vi "AlGaInPAs_v20b.vi"(2 "Debug Mode":bool, 3 "Elapsed Time(s)":dbl, 4 "State":enum16{"Edit", "Start", "Run", "End", "Idle"}(ring), 5 "Argument List In":string[](array[string])) -> (0 "Status Out":string, 1 "Argument List Out":string[](array[string]))   [LabVIEW 2011]
panel:
  out "source ref array":refnum<vi>[](array[refnum])
  in  "Se bubbler":T1={"Active"=FALSE, "Prep"=FALSE, "Run"=FALSE, "Flow"=0.0, "Dilution"=FALSE, "Calculated"=0, "MFC1 flow"=0.0, "MFC2 flow"=10.0, "MFC3 flow"=100.0} caption="Al" {"MFC1 flow" format="%.4f"; "MFC3 flow" format="%.1f"; "MFC2 flow" format="%.2f"; "Calculated" items=["Flow", "MFC1", "MFC2", "MFC3"]; "Flow" format="%.2f"}
  in  "P bubbler":T2 caption="Al" {"Flow" format="%.2f"}
  in  "As gas":T2 caption="Al" {"Flow" format="%.2f"}
  in  "P gas":T2 caption="Al" {"Flow" format="%.2f"}
  in  "In bubbler":T2 caption="Al" {"Flow" format="%.2f"}
  in  "Ga bubbler":T1={"Active"=FALSE, "Prep"=FALSE, "Run"=FALSE, "Flow"=0.0, "Dilution"=FALSE, "Calculated"=0, "MFC1 flow"=0.0, "MFC2 flow"=10.0, "MFC3 flow"=100.0} caption="Al" {"MFC1 flow" format="%.4f"; "MFC3 flow" format="%.1f"; "MFC2 flow" format="%.2f"; "Calculated" items=["Flow", "MFC1", "MFC2", "MFC3"]; "Flow" format="%.2f"}
  in  "Al bubbler":T2 caption="Al" {"Flow" format="%.2f"}
  in  "Tab Control":T3(tab)
  out "Al Prep":bool caption="Pre-run"
  out "Al Run":bool caption="Run"
  out "Al Flow":dbl caption="Al Flow (0-100 sscm)" format="%.2f"
  out "Ga MFC1 flow":dbl caption="R1 (0-10 sscm)" format="%.4f"
  out "Ga MFC3 flow":dbl=100.0 caption="R3 (0-1000 sscm)" format="%.1f"
  out "Ga MFC2 flow":dbl=10.0 caption="R2 (0-100 sscm)" format="%.2f"
  out "Ga Calculated":u16(ring)=1 caption="Calculated" items=["Ga flow", "MFC1", "MFC2", "MFC3"]
  out "Ga Dilution":bool caption="Dilute"
  out "Ga Prep":bool caption="Pre-run"
  out "Ga Run":bool caption="Run"
  out "Ga Flow":dbl caption="Ga Flow (0-10 sscm)" format="%.2f"
  out "In Prep":bool caption="Pre-run"
  out "In Run":bool caption="Run"
  out "In Flow":dbl caption="In Flow (0-100 sscm)" format="%.2f"
  out "P gas Run":bool caption="Run"
  out "P gas Prep":bool caption="Pre-run"
  out "P gas Flow":dbl caption="PH3 Flow (0-100 sscm)" format="%.2f"
  out "As gas Prep":bool caption="Pre-run"
  out "As gas Run":bool caption="Run"
  out "As gas Flow":dbl caption="AsH3 Flow (0-10 sscm)" format="%.2f"
  out "P liq Prep":bool caption="Pre-run"
  out "P liq Run":bool caption="Run"
  out "P liq Flow":dbl caption="P bubbler Flow (0-100 sscm)" format="%.2f"
  out "Se MFC1 flow":dbl caption="R1 (0-10 sscm)" format="%.4f"
  out "Se MFC3 flow":dbl=100.0 caption="R3 (0-1000 sscm)" format="%.1f"
  out "Se MFC2 flow":dbl=10.0 caption="R2 (0-100 sscm)" format="%.2f"
  out "Se Calculated":u16(ring)=1 caption="Calculated" items=["Ga flow", "MFC1", "MFC2", "MFC3"]
  out "Se Dilution":bool caption="Dilute"
  out "Se Prep":bool caption="Pre-run"
  out "Se Run":bool caption="Run"
  out "Se Flow":dbl caption="Se Flow (0-10 sscm)" format="%.2f"
  out "prep_done":bool
  out "run started":bool
  out "first":bool=TRUE
  out "total time":dbl
  out "is OK?":bool
  in  "prep_time":dbl
  in  "Cancel":bool
  in  "OK":bool
  out "tTotal(s) 2":dbl
  # "s"
  # "Add pre-run time to run time in editor."
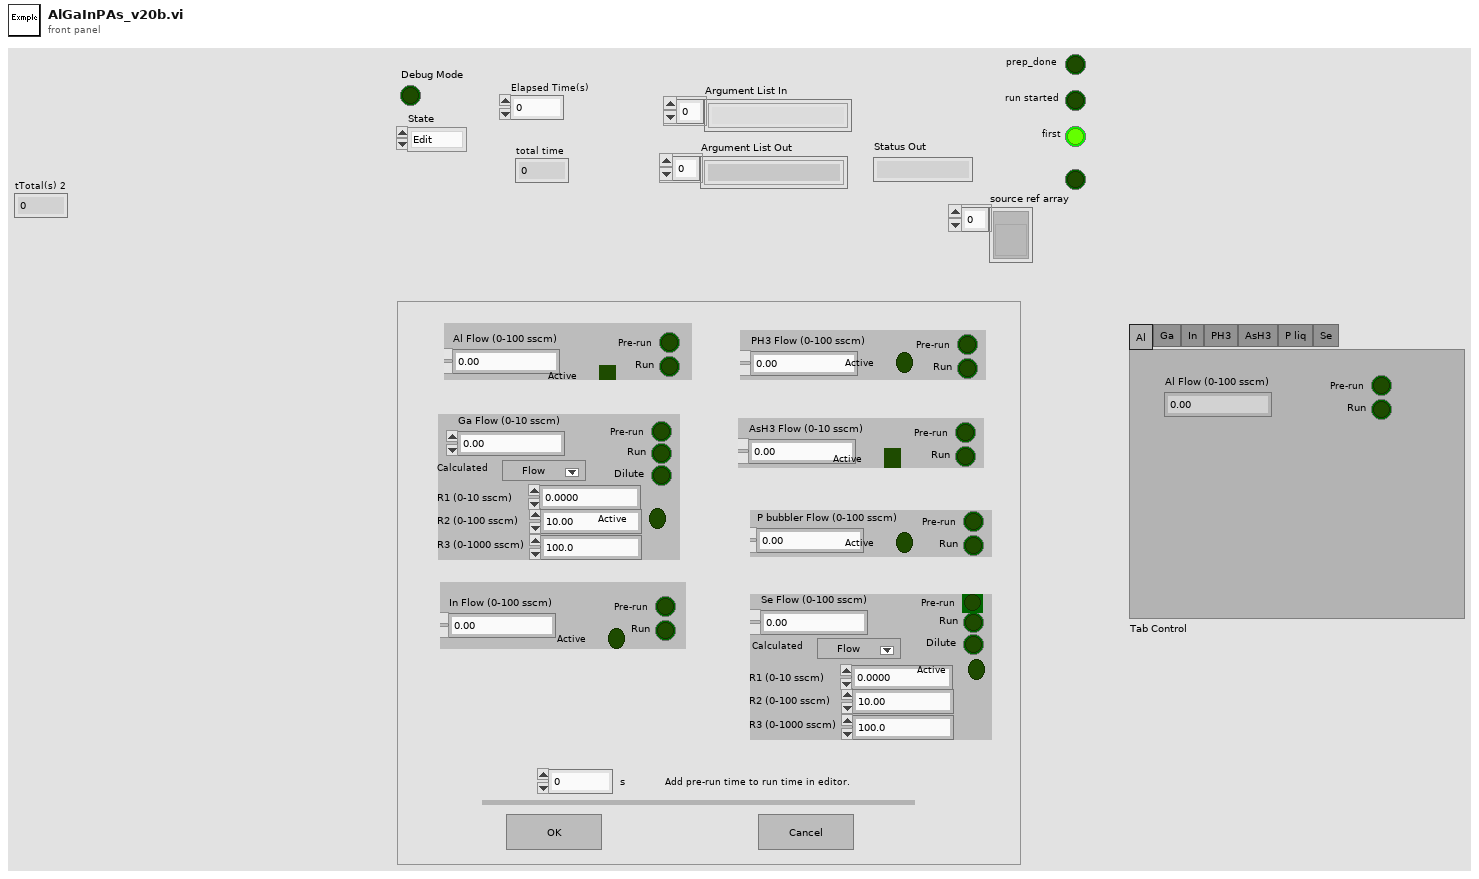
[diagram p1: front panel]
types:
  T1 = cluster{"Active":bool, "Prep":bool, "Run":bool, "Flow":dbl, "Dilution":bool, "Calculated":u16, "MFC1 flow":dbl, "MFC2 flow":dbl, "MFC3 flow":dbl}
  T2 = cluster{"Active":bool, "Prep":bool, "Run":bool, "Flow":dbl}
  T3 = enum32{"Al", "Ga", "In", "PH3", "AsH3", "P liq", "Se"}
  T4 = enum16{"Discrete", "Continuous", "Instantaneous", "Finite"}
  T5 = enum32{"Invalid", "Default", "Floating", "Floating/Auto-Hide", "Modal"}
  T6 = enum8{"Enabled", "Disabled", "Disabled and Grayed Out"}
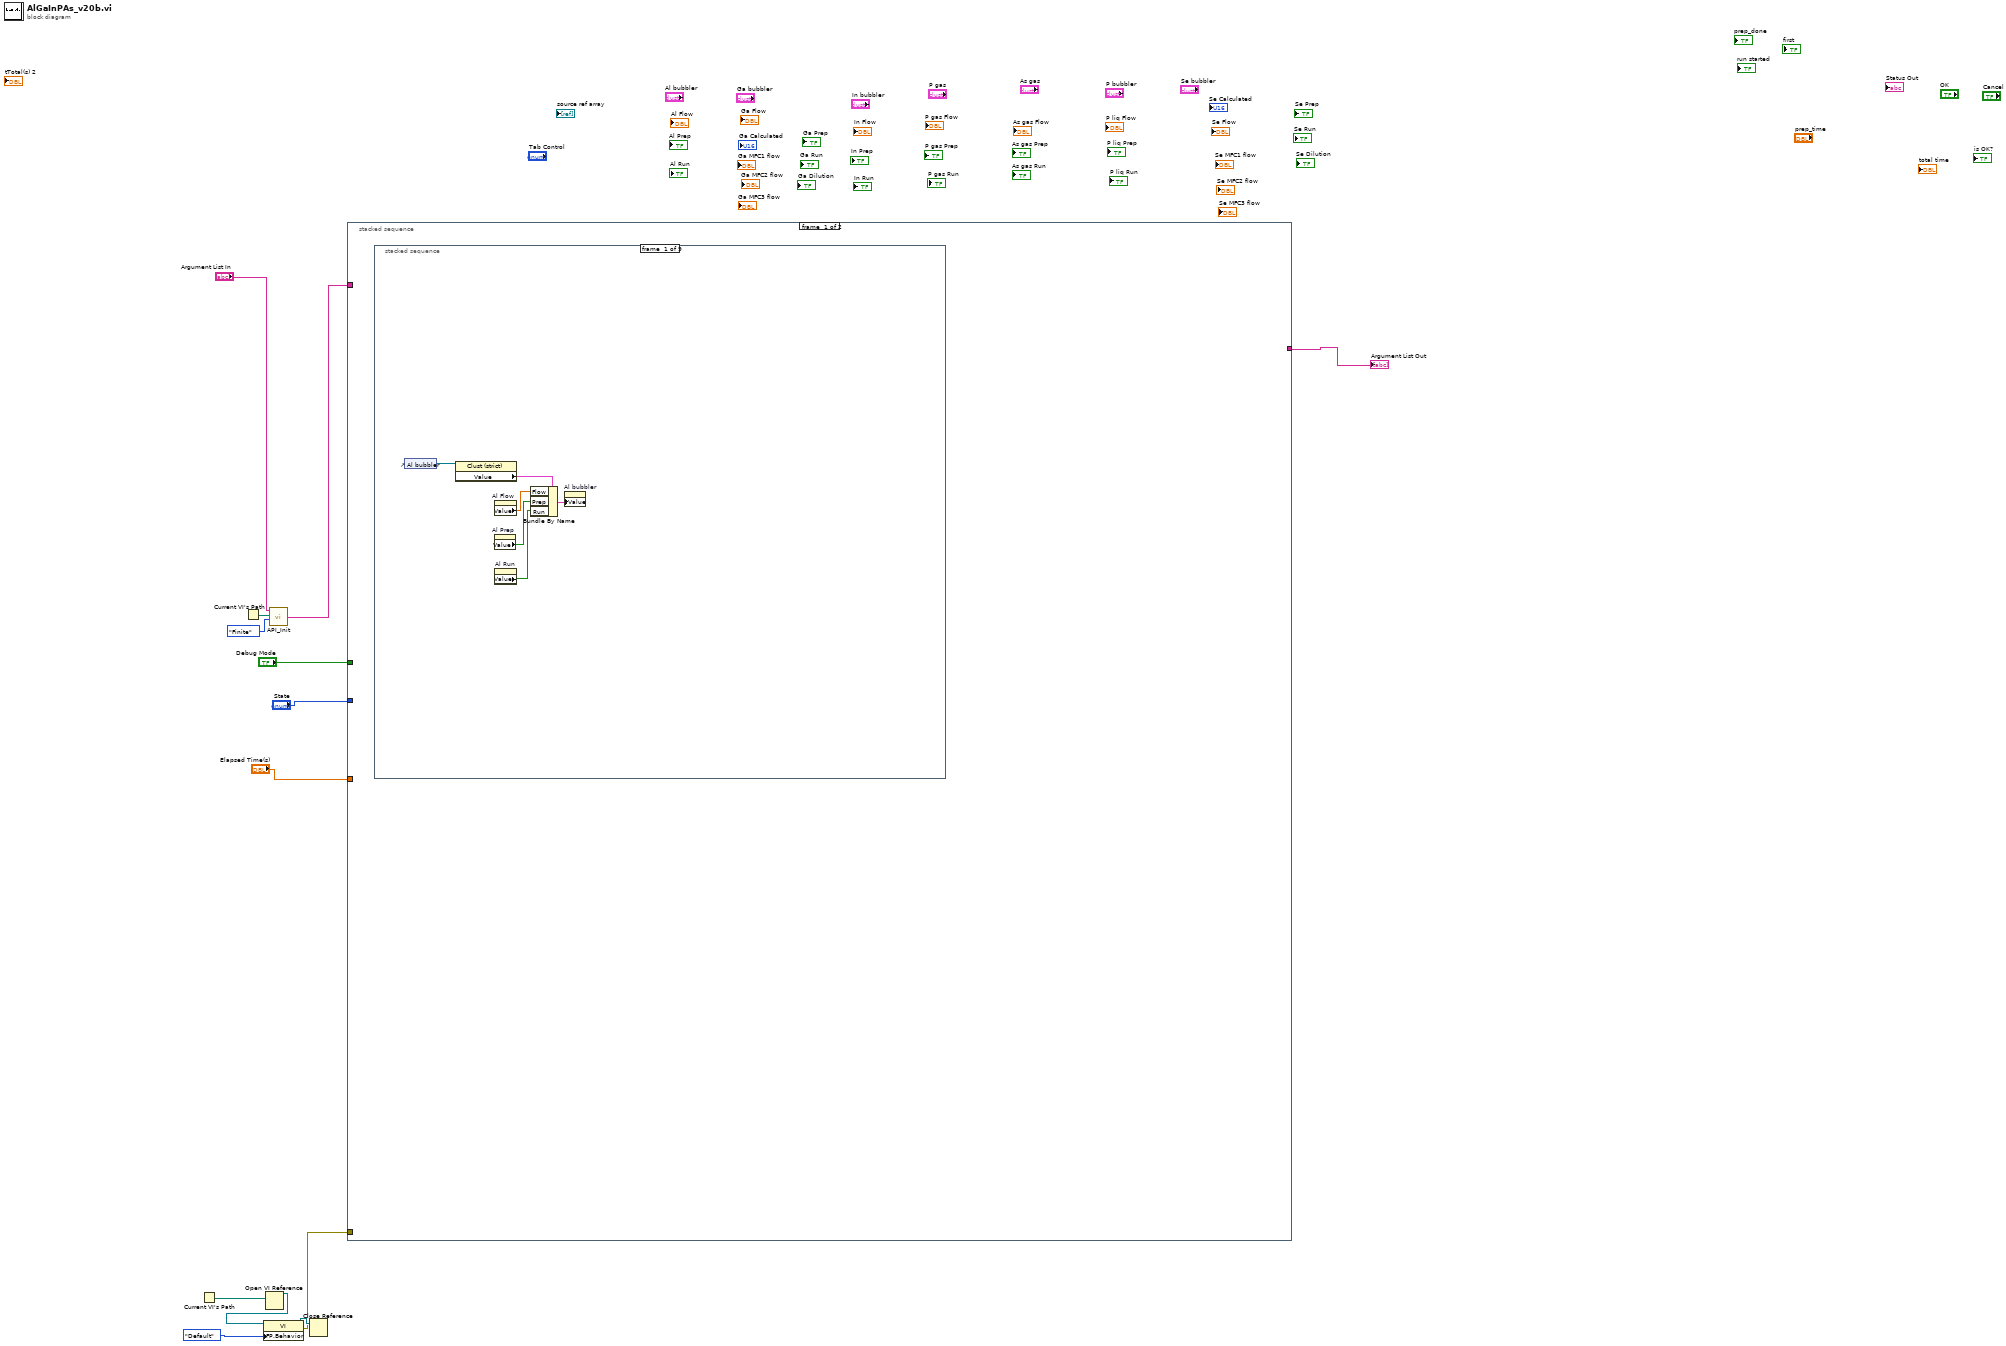
[diagram p0: block diagram]
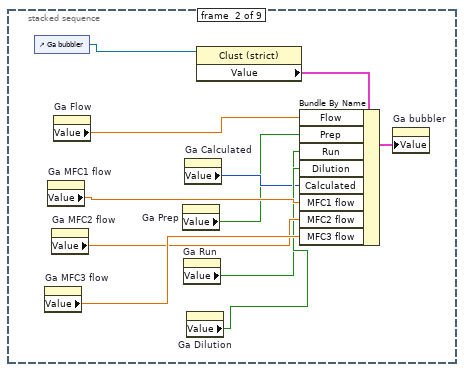
[diagram p2: hidden frame]
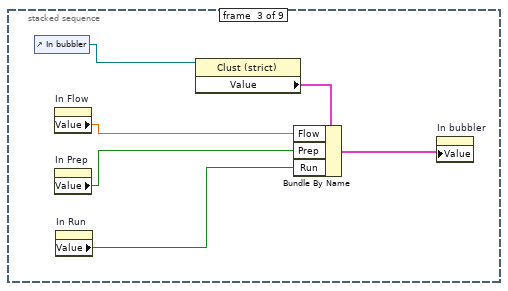
[diagram p3: hidden frame]
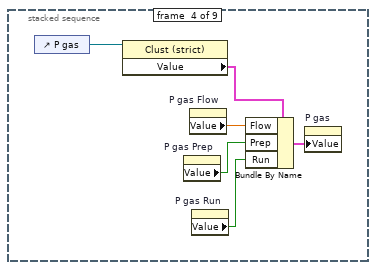
[diagram p4: hidden frame]
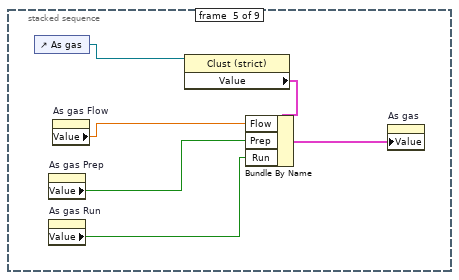
[diagram p5: hidden frame]
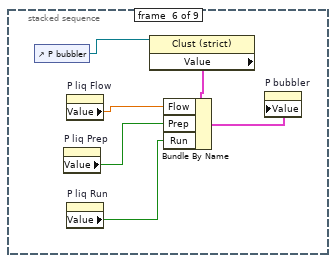
[diagram p6: hidden frame]
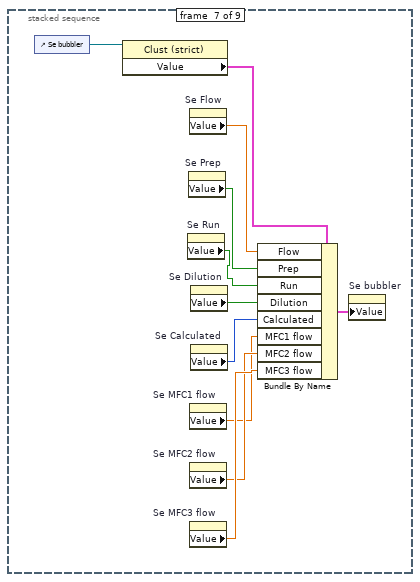
[diagram p7: hidden frame]
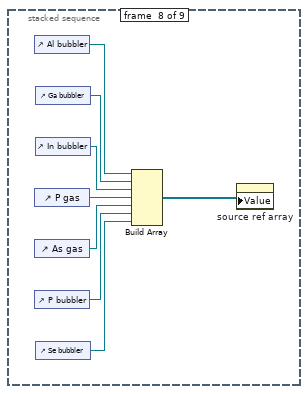
[diagram p8: hidden frame]
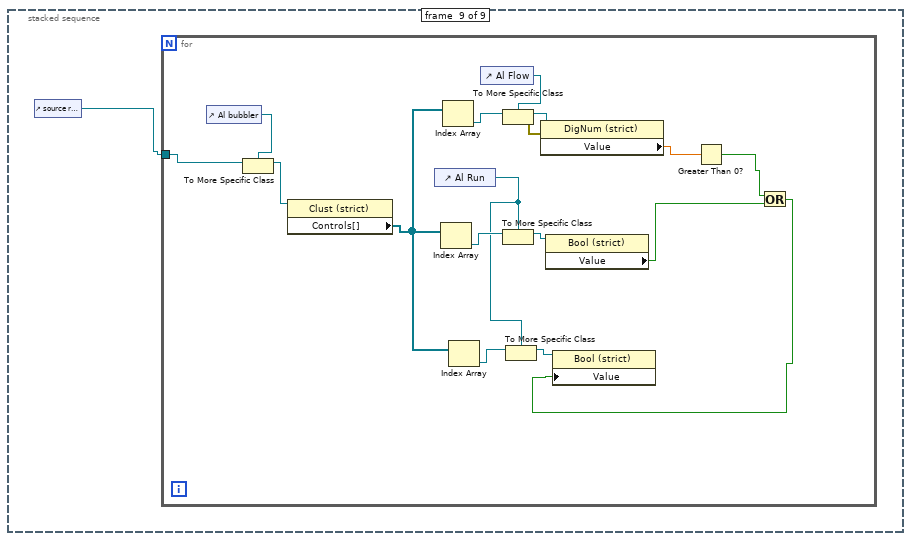
[diagram p9: hidden frame]
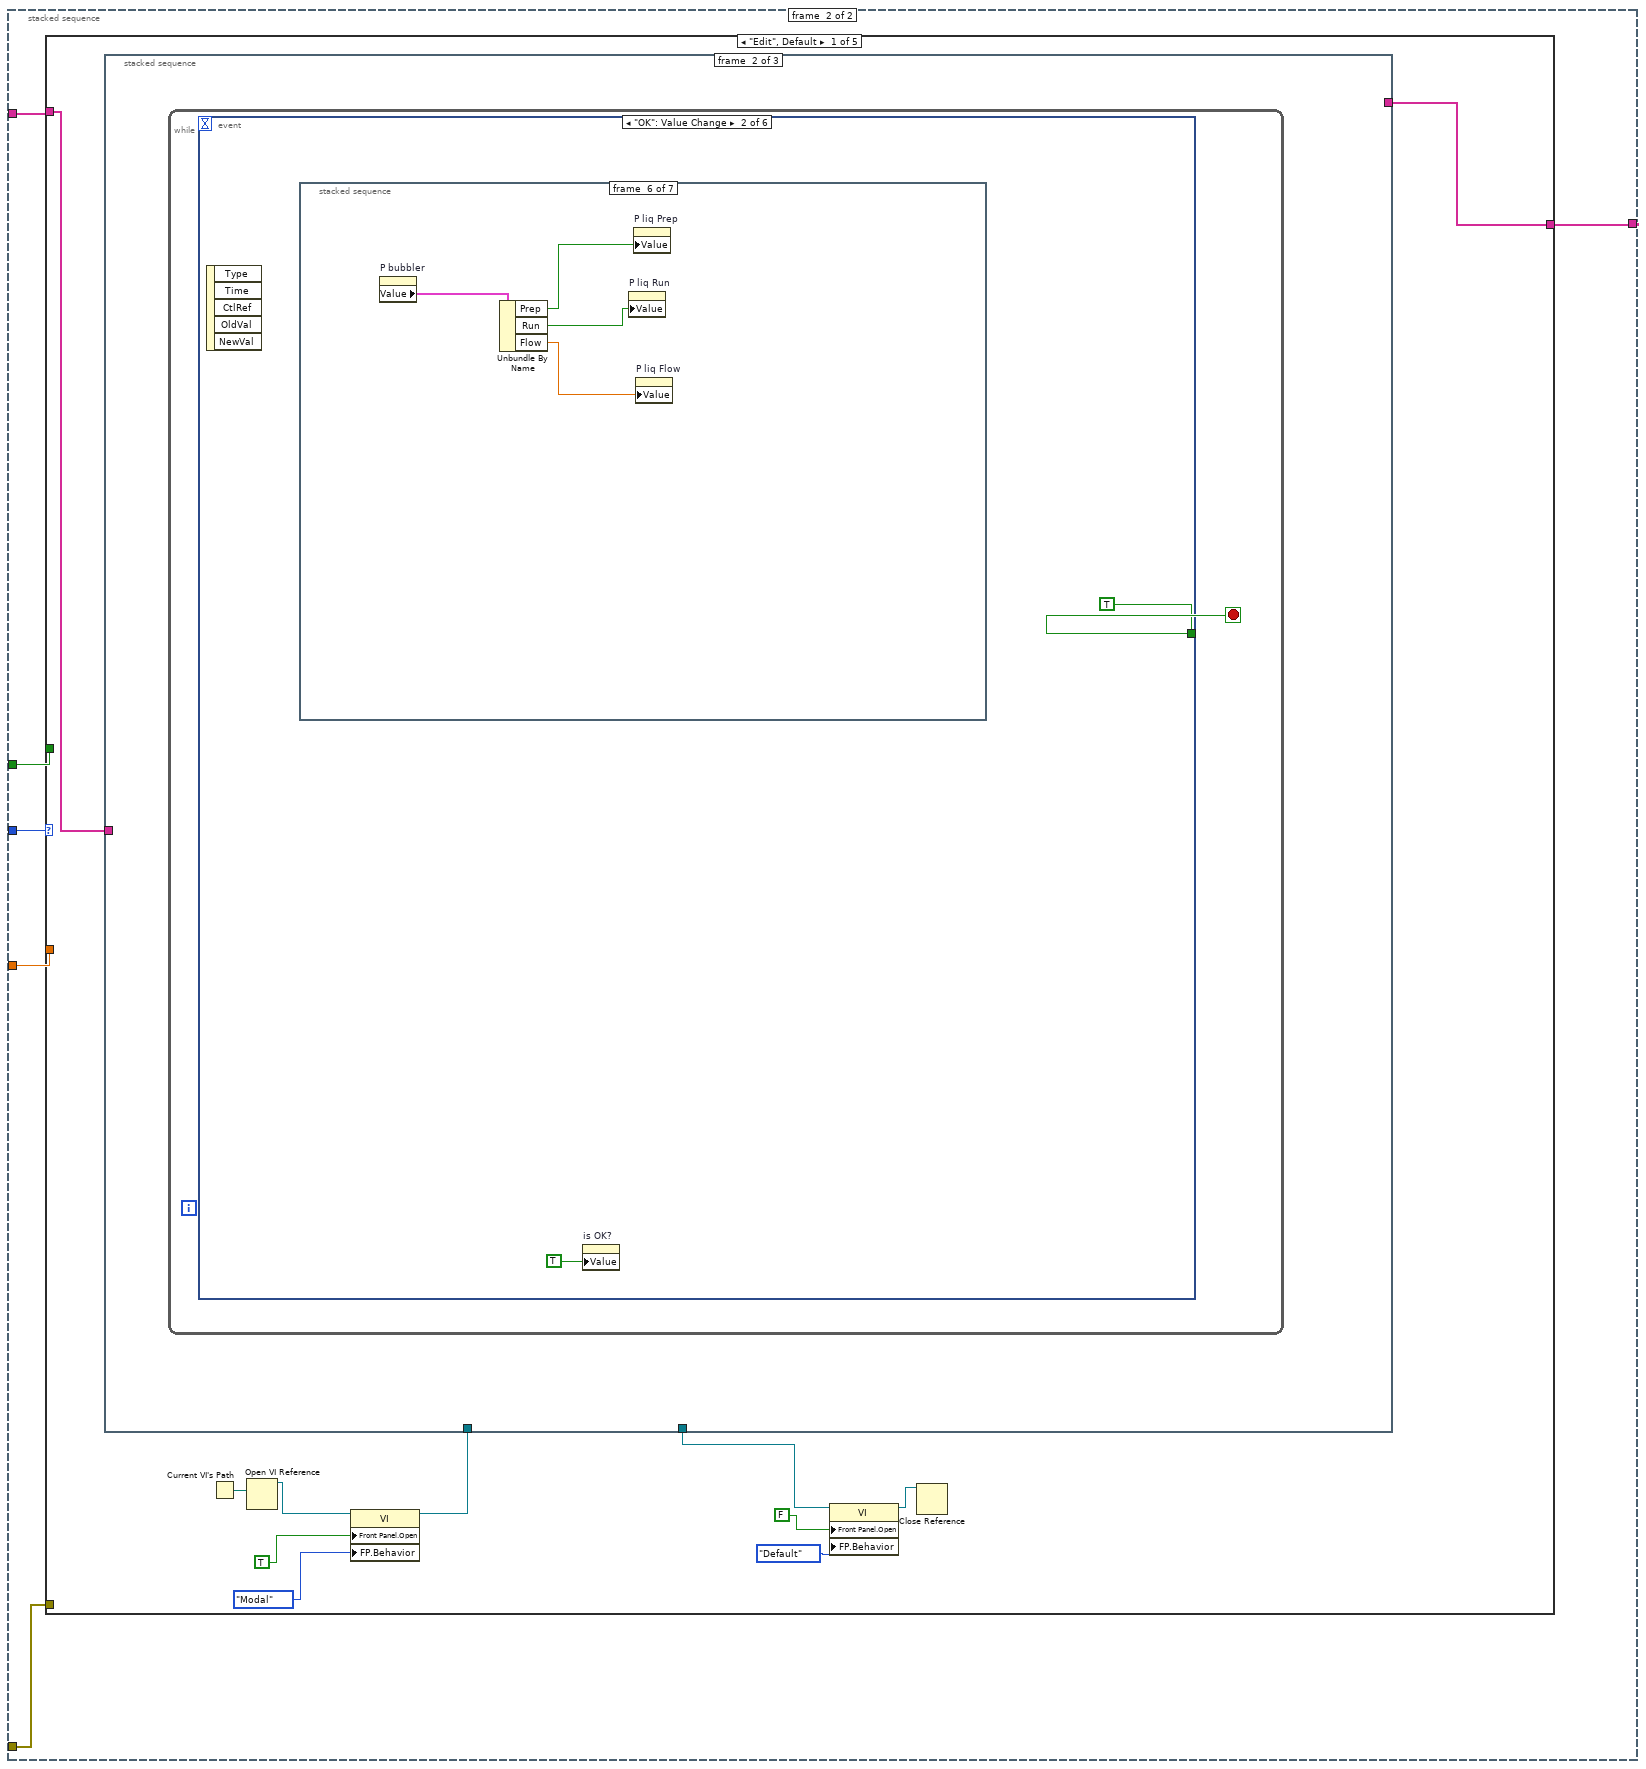
[diagram p10: hidden frame]
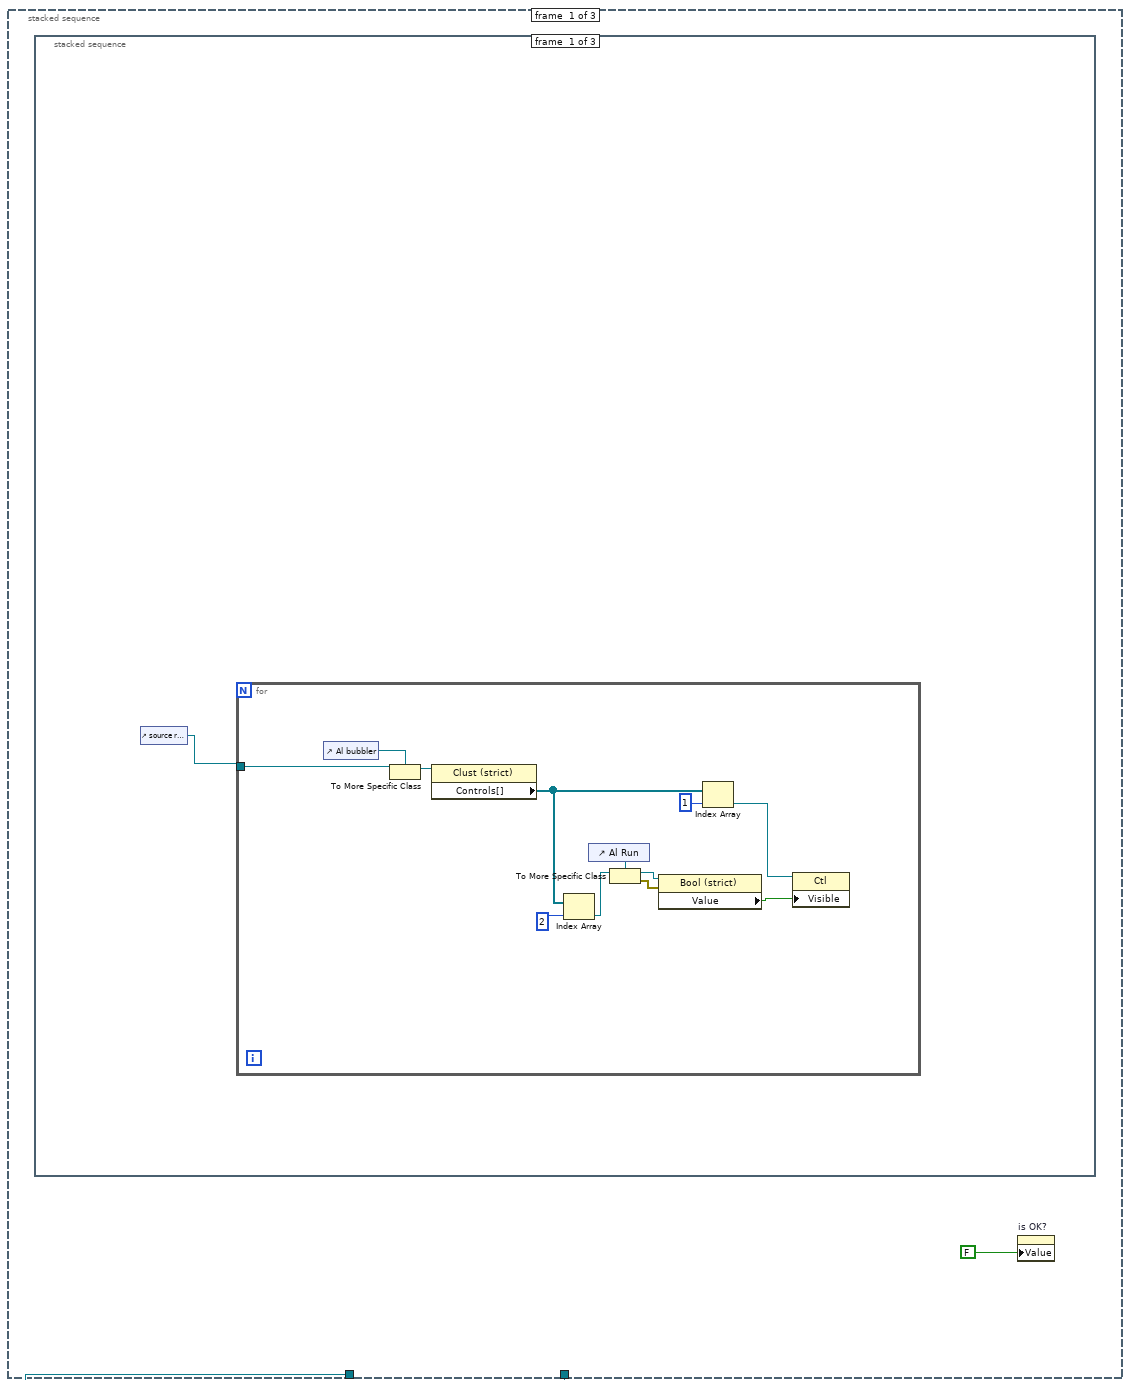
[diagram p11: hidden frame]
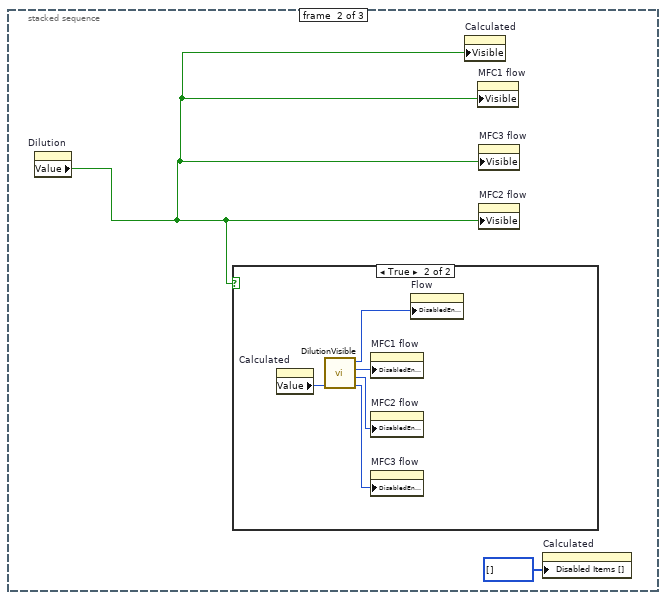
[diagram p12: hidden frame]
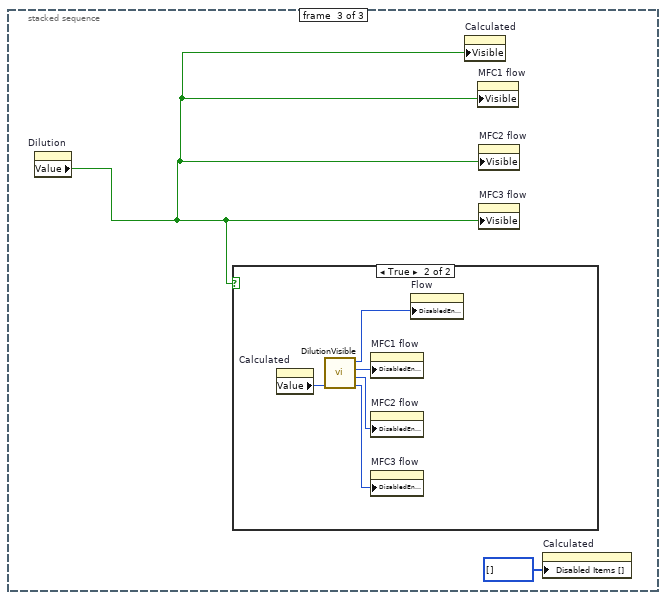
[diagram p14: hidden frame]
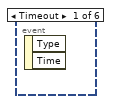
[diagram p16: hidden frame]
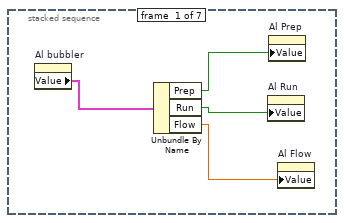
[diagram p17: hidden frame]
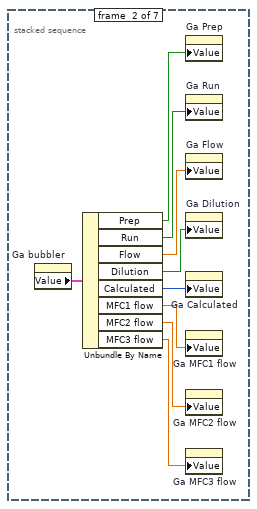
[diagram p18: hidden frame]
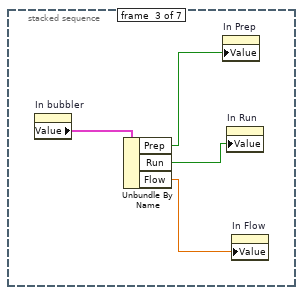
[diagram p19: hidden frame]
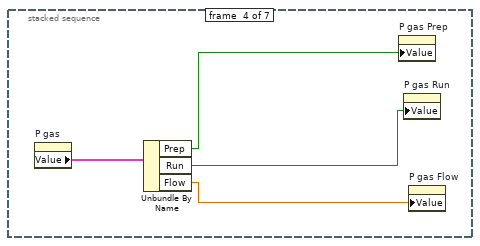
[diagram p20: hidden frame]
diagram:
  n1 = Current VI's Path() -> (path=w9:path)
  n2 = Current VI's Path() -> (path=w4:path)
  n3 = Open VI Reference(vi path=w9) -> (vi reference=w8:refnum<vi>)  [unwired: 1 in, 5 out]
  n4 = property class="VI"(reference=w8, "FP.Behavior"=T5."Default" ("Front Panel Window:Behavior")) -> (reference out=w6:refnum<vi>, error out=w5:errorcluster)  [unwired: 1 in]
  n5 = call "API_Init.vi"("API Mode"=T4."Finite", "VI Path"=w4, "Argument List In"="Argument List In") -> ("Argument List Out"=w1:string[])  [unwired: 1 in]
  n6 = Close Reference(reference=w6) -> ()  [unwired: 1 in, 1 out]
  n7 = stacked-sequence {
    tunnel: "State" -> [_ w97]
    tunnel: "Debug Mode" -> [_ w96]
    tunnel: "Elapsed Time(s)" -> [_ w95]
    tunnel: [_ w94] -> w10
    tunnel: w5 -> [_ w93]
    tunnel: w1 -> [_ w92]
    frame #0 {
      n8 = stacked-sequence {
        frame #0 {
          n9 = control-ref of="Al bubbler"() -> (w19:refnum<vi>)
          n10 = property class="Clust (strict)"(reference=w19) -> ("Value"=w18:T2)  [unwired: 1 in, 2 out]
          n11 = property on="Al Prep" class="Bool (strict)"() -> ("Value"=w16:bool)  [unwired: 2 in, 2 out]
          n12 = property on="Al Flow" class="DigNum (strict)"() -> ("Value"=w17:dbl)  [unwired: 2 in, 2 out]
          n13 = property on="Al Run" class="Bool (strict)"() -> ("Value"=w15:bool)  [unwired: 2 in, 2 out]
          n14 = Bundle By Name(cluster=w18, "Flow"=w17, "Prep"=w16, "Run"=w15) -> (w14:T2)
          n15 = property on="Al bubbler" class="Clust (strict)"("Value"=w14) -> ()  [unwired: 2 in, 2 out]
        }
        frame #1 {
          n16 = control-ref of="Ga bubbler"() -> (w20:refnum<vi>)
          n17 = property on="Ga MFC3 flow" class="DigNum (strict)"() -> ("Value"=w30:dbl)  [unwired: 2 in, 2 out]
          n18 = property on="Ga MFC1 flow" class="DigNum (strict)"() -> ("Value"=w28:dbl)  [unwired: 2 in, 2 out]
          n19 = property on="Ga MFC2 flow" class="DigNum (strict)"() -> ("Value"=w29:dbl)  [unwired: 2 in, 2 out]
          n20 = property on="Ga Flow" class="DigNum (strict)"() -> ("Value"=w23:dbl)  [unwired: 2 in, 2 out]
          n21 = property on="Ga Prep" class="Bool (strict)"() -> ("Value"=w24:bool)  [unwired: 2 in, 2 out]
          n22 = property on="Ga Run" class="Bool (strict)"() -> ("Value"=w26:bool)  [unwired: 2 in, 2 out]
          n23 = property on="Ga Calculated" class="Ring (strict)"() -> ("Value"=w25:u16)  [unwired: 2 in, 2 out]
          n24 = property on="Ga Dilution" class="Bool (strict)"() -> ("Value"=w27:bool)  [unwired: 2 in, 2 out]
          n25 = property class="Clust (strict)"(reference=w20) -> ("Value"=w21:T1)  [unwired: 1 in, 2 out]
          n26 = Bundle By Name(cluster=w21, "Flow"=w23, "Prep"=w24, "Run"=w26, "Dilution"=w27, "Calculated"=w25, "MFC1 flow"=w28, "MFC2 flow"=w29, "MFC3 flow"=w30) -> (w22:T1)
          n27 = property on="Ga bubbler" class="Clust (strict)"("Value"=w22) -> ()  [unwired: 2 in, 2 out]
        }
        frame #2 {
          n28 = control-ref of="In bubbler"() -> (w31:refnum<vi>)
          n29 = property on="In Flow" class="DigNum (strict)"() -> ("Value"=w33:dbl)  [unwired: 2 in, 2 out]
          n30 = property on="In Prep" class="Bool (strict)"() -> ("Value"=w35:bool)  [unwired: 2 in, 2 out]
          n31 = property on="In Run" class="Bool (strict)"() -> ("Value"=w36:bool)  [unwired: 2 in, 2 out]
          n32 = property class="Clust (strict)"(reference=w31) -> ("Value"=w32:T2)  [unwired: 1 in, 2 out]
          n33 = Bundle By Name(cluster=w32, "Flow"=w33, "Prep"=w35, "Run"=w36) -> (w34:T2)
          n34 = property on="In bubbler" class="Clust (strict)"("Value"=w34) -> ()  [unwired: 2 in, 2 out]
        }
        frame #3 {
          n35 = control-ref of="P gas"() -> (w37:refnum<vi>)
          n36 = property class="Clust (strict)"(reference=w37) -> ("Value"=w38:T2)  [unwired: 1 in, 2 out]
          n37 = property on="P gas Prep" class="Bool (strict)"() -> ("Value"=w41:bool)  [unwired: 2 in, 2 out]
          n38 = property on="P gas Flow" class="DigNum (strict)"() -> ("Value"=w39:dbl)  [unwired: 2 in, 2 out]
          n39 = property on="P gas Run" class="Bool (strict)"() -> ("Value"=w42:bool)  [unwired: 2 in, 2 out]
          n40 = Bundle By Name(cluster=w38, "Flow"=w39, "Prep"=w41, "Run"=w42) -> (w40:T2)
          n41 = property on="P gas" class="Clust (strict)"("Value"=w40) -> ()  [unwired: 2 in, 2 out]
        }
        frame #4 {
          n42 = control-ref of="As gas"() -> (w44:refnum<vi>)
          n43 = property on="As gas Prep" class="Bool (strict)"() -> ("Value"=w47:bool)  [unwired: 2 in, 2 out]
          n44 = property on="As gas Run" class="Bool (strict)"() -> ("Value"=w48:bool)  [unwired: 2 in, 2 out]
          n45 = property on="As gas Flow" class="DigNum (strict)"() -> ("Value"=w46:dbl)  [unwired: 2 in, 2 out]
          n46 = property class="Clust (strict)"(reference=w44) -> ("Value"=w43:T2)  [unwired: 1 in, 2 out]
          n47 = Bundle By Name(cluster=w43, "Flow"=w46, "Prep"=w47, "Run"=w48) -> (w45:T2)
          n48 = property on="As gas" class="Clust (strict)"("Value"=w45) -> ()  [unwired: 2 in, 2 out]
        }
        frame #5 {
          n49 = control-ref of="P bubbler"() -> (w49:refnum<vi>)
          n50 = property on="P liq Prep" class="Bool (strict)"() -> ("Value"=w53:bool)  [unwired: 2 in, 2 out]
          n51 = property on="P liq Flow" class="DigNum (strict)"() -> ("Value"=w52:dbl)  [unwired: 2 in, 2 out]
          n52 = property on="P liq Run" class="Bool (strict)"() -> ("Value"=w54:bool)  [unwired: 2 in, 2 out]
          n53 = property class="Clust (strict)"(reference=w49) -> ("Value"=w50:T2)  [unwired: 1 in, 2 out]
          n54 = Bundle By Name(cluster=w50, "Flow"=w52, "Prep"=w53, "Run"=w54) -> (w51:T2)
          n55 = property on="P bubbler" class="Clust (strict)"("Value"=w51) -> ()  [unwired: 2 in, 2 out]
        }
        frame #6 {
          n56 = control-ref of="Se bubbler"() -> (w55:refnum<vi>)
          n57 = property class="Clust (strict)"(reference=w55) -> ("Value"=w56:T1)  [unwired: 1 in, 2 out]
          n58 = property on="Se Run" class="Bool (strict)"() -> ("Value"=w60:bool)  [unwired: 2 in, 2 out]
          n59 = property on="Se Prep" class="Bool (strict)"() -> ("Value"=w59:bool)  [unwired: 2 in, 2 out]
          n60 = property on="Se Flow" class="DigNum (strict)"() -> ("Value"=w58:dbl)  [unwired: 2 in, 2 out]
          n61 = property on="Se MFC1 flow" class="DigNum (strict)"() -> ("Value"=w63:dbl)  [unwired: 2 in, 2 out]
          n62 = property on="Se MFC2 flow" class="DigNum (strict)"() -> ("Value"=w64:dbl)  [unwired: 2 in, 2 out]
          n63 = property on="Se MFC3 flow" class="DigNum (strict)"() -> ("Value"=w65:dbl)  [unwired: 2 in, 2 out]
          n64 = property on="Se Dilution" class="Bool (strict)"() -> ("Value"=w61:bool)  [unwired: 2 in, 2 out]
          n65 = property on="Se Calculated" class="Ring (strict)"() -> ("Value"=w62:u16)  [unwired: 2 in, 2 out]
          n66 = Bundle By Name(cluster=w56, "Flow"=w58, "Prep"=w59, "Run"=w60, "Dilution"=w61, "Calculated"=w62, "MFC1 flow"=w63, "MFC2 flow"=w64, "MFC3 flow"=w65) -> (w57:T1)
          n67 = property on="Se bubbler" class="Clust (strict)"("Value"=w57) -> ()  [unwired: 2 in, 2 out]
        }
        frame #7 {
          n68 = control-ref of="Al bubbler"() -> (w73:refnum<vi>)
          n69 = control-ref of="P gas"() -> (w70:refnum<vi>)
          n70 = control-ref of="As gas"() -> (w69:refnum<vi>)
          n71 = control-ref of="P bubbler"() -> (w68:refnum<vi>)
          n72 = control-ref of="Ga bubbler"() -> (w72:refnum<vi>)
          n73 = control-ref of="In bubbler"() -> (w71:refnum<vi>)
          n74 = control-ref of="Se bubbler"() -> (w67:refnum<vi>)
          n75 = Build Array(w73, w72, w71, w70, w69, w68, w67) -> (w66:refnum<vi>[])
          n76 = property on="source ref array" class="Arr (strict)"("Value"=w66) -> ()  [unwired: 2 in, 2 out]
        }
        frame #8 {
          n77 = control-ref of="source ref array"() -> (w74:refnum<vi>)
          n78 = for {
            tunnel: w74 -> [w90]
            n79 = control-ref of="Al bubbler"() -> (w89:refnum<vi>)
            n80 = To More Specific Class(target class=w89, reference=w90) -> (specific class reference=w88:refnum<vi>)  [unwired: 1 in, 1 out]
            n81 = property class="Clust (strict)"(reference=w88) -> ("Controls[]"=w87:refnum<vi>[])  [unwired: 1 in, 2 out]
            n82 = control-ref of="Al Run"() -> (w84:refnum<vi>)
            n83 = Index Array(array=w87) -> (element=w86:refnum<vi>)  [unwired: 1 in]
            n84 = Index Array(array=w87) -> (element=w83:refnum<vi>)  [unwired: 1 in]
            n85 = Index Array(array=w87) -> (element=w85:refnum<vi>)  [unwired: 1 in]
            n86 = control-ref of="Al Flow"() -> (w82:refnum<vi>)
            n87 = To More Specific Class(target class=w82, reference=w83) -> (specific class reference=w79:refnum<vi>, error out=w78:errorcluster)  [unwired: 1 in]
            n88 = To More Specific Class(target class=w84, reference=w86) -> (specific class reference=w81:refnum<vi>)  [unwired: 1 in, 1 out]
            n89 = To More Specific Class(target class=w84, reference=w85) -> (specific class reference=w80:refnum<vi>)  [unwired: 1 in, 1 out]
            n90 = property class="DigNum (strict)"(reference=w79, error in=w78) -> ("Value"=w77:dbl)  [unwired: 2 out]
            n91 = property class="Bool (strict)"(reference=w81) -> ("Value"=w76:bool)  [unwired: 1 in, 2 out]
            n92 = Greater Than 0?(x=w77) -> (x > 0?=w91:bool)
            n93 = Or(x=w91, y=w76) -> (x .or. y?=w75:bool)
            n94 = property class="Bool (strict)"(reference=w80, "Value"=w75) -> ()  [unwired: 1 in, 2 out]
          }
        }
      }
    }
    frame #1 {
      n95 = case shown="\"Edit\", Default" w97 {
        tunnel: w96 -> [_ w235 w247 _ _]
        tunnel: w95 -> [_ _ w248 _ _]
        tunnel: w92 -> [w99 w240 w246 w343 w344]
        tunnel: [w98 w239 w245 w343 w344] -> w94
        tunnel: w93 -> [_ _ _ _ _]
        frame "Edit", Default {
          n96 = Current VI's Path() -> (path=w104:path)
          n97 = Open VI Reference(vi path=w104) -> (vi reference=w103:refnum<vi>)  [unwired: 1 in, 5 out]
          n98 = property class="VI"(reference=w103, "Front Panel.Open"=TRUE ("Front Panel Window:Open"), "FP.Behavior"=T5."Modal" ("Front Panel Window:Behavior")) -> (reference out=w102:refnum<vi>)  [unwired: 1 in, 1 out]
          n99 = stacked-sequence {
            tunnel: w99 -> [_ _ w230]
            tunnel: w102 -> [w110 _ _]
            tunnel: [w110 _ _] -> w106
            tunnel: [_ _ w231] -> w98
            frame #0 {
              n100 = stacked-sequence {
                frame #0 {
                  n101 = control-ref of="source ref array"() -> (w111:refnum<vi>)
                  n102 = for {
                    tunnel: w111 -> [w123]
                    n103 = control-ref of="Al bubbler"() -> (w122:refnum<vi>)
                    n104 = To More Specific Class(target class=w122, reference=w123) -> (specific class reference=w119:refnum<vi>)  [unwired: 1 in, 1 out]
                    n105 = property class="Clust (strict)"(reference=w119) -> ("Controls[]"=w118:refnum<vi>[])  [unwired: 1 in, 2 out]
                    n106 = Index Array(array=w118, index=2) -> (element=w115:refnum<vi>)
                    n107 = control-ref of="Al Run"() -> (w116:refnum<vi>)
                    n108 = To More Specific Class(target class=w116, reference=w115) -> (specific class reference=w114:refnum<vi>, error out=w113:errorcluster)  [unwired: 1 in]
                    n109 = property class="Bool (strict)"(reference=w114, error in=w113) -> ("Value"=w112:bool)  [unwired: 2 out]
                    n110 = Index Array(array=w118, index=1) -> (element=w120:refnum<vi>)
                    n111 = property class="Ctl"(reference=w120, "Visible"=w112) -> ()  [unwired: 1 in, 2 out]
                  }
                }
                frame #1 {
                  n112 = property on="Dilution" class="Bool (strict)"() -> ("Value"=w125:bool)  [unwired: 2 in, 2 out]
                  n113 = case shown="True" w125 {
                    frame False {
                    }
                    frame True {
                      n114 = property on="Calculated" class="Ring (strict)"() -> ("Value"=w126:u16)  [unwired: 2 in, 2 out]
                      n115 = call "DilutionVisible.vi"("calculated"=w126) -> ("MFC3"=w129:u16, "MFC2"=w128:u16, "MFC1"=w127:u16, "flow"=w130:u16)  [unwired: 3 in]
                      n116 = property on="MFC1 flow" class="DigNum (strict)"("DisabledEnum"=w127) -> ()  [unwired: 2 in, 2 out]
                      n117 = property on="MFC2 flow" class="DigNum (strict)"("DisabledEnum"=w128) -> ()  [unwired: 2 in, 2 out]
                      n118 = property on="MFC3 flow" class="DigNum (strict)"("DisabledEnum"=w129) -> ()  [unwired: 2 in, 2 out]
                      n119 = property on="Flow" class="DigNum (strict)"("DisabledEnum"=w130) -> ()  [unwired: 2 in, 2 out]
                    }
                  }
                  n120 = property on="Calculated" class="Ring (strict)"("Visible"=w125) -> ()  [unwired: 2 in, 2 out]
                  n121 = property on="MFC1 flow" class="DigNum (strict)"("Visible"=w125) -> ()  [unwired: 2 in, 2 out]
                  n122 = property on="MFC3 flow" class="DigNum (strict)"("Visible"=w125) -> ()  [unwired: 2 in, 2 out]
                  n123 = property on="MFC2 flow" class="DigNum (strict)"("Visible"=w125) -> ()  [unwired: 2 in, 2 out]
                  n124 = property on="Calculated" class="Ring (strict)"("Disabled Items []"=i32[] []) -> ()  [unwired: 2 in, 2 out]
                }
                frame #2 {
                  n125 = property on="Dilution" class="Bool (strict)"() -> ("Value"=w132:bool)  [unwired: 2 in, 2 out]
                  n126 = case shown="True" w132 {
                    frame False {
                    }
                    frame True {
                      n127 = property on="Calculated" class="Ring (strict)"() -> ("Value"=w133:u16)  [unwired: 2 in, 2 out]
                      n128 = call "DilutionVisible.vi"("calculated"=w133) -> ("MFC3"=w136:u16, "MFC2"=w135:u16, "MFC1"=w134:u16, "flow"=w137:u16)  [unwired: 3 in]
                      n129 = property on="MFC1 flow" class="DigNum (strict)"("DisabledEnum"=w134) -> ()  [unwired: 2 in, 2 out]
                      n130 = property on="MFC2 flow" class="DigNum (strict)"("DisabledEnum"=w135) -> ()  [unwired: 2 in, 2 out]
                      n131 = property on="MFC3 flow" class="DigNum (strict)"("DisabledEnum"=w136) -> ()  [unwired: 2 in, 2 out]
                      n132 = property on="Flow" class="DigNum (strict)"("DisabledEnum"=w137) -> ()  [unwired: 2 in, 2 out]
                    }
                  }
                  n133 = property on="Calculated" class="Ring (strict)"("Visible"=w132) -> ()  [unwired: 2 in, 2 out]
                  n134 = property on="MFC1 flow" class="DigNum (strict)"("Visible"=w132) -> ()  [unwired: 2 in, 2 out]
                  n135 = property on="MFC2 flow" class="DigNum (strict)"("Visible"=w132) -> ()  [unwired: 2 in, 2 out]
                  n136 = property on="MFC3 flow" class="DigNum (strict)"("Visible"=w132) -> ()  [unwired: 2 in, 2 out]
                  n137 = property on="Calculated" class="Ring (strict)"("Disabled Items []"=i32[] []) -> ()  [unwired: 2 in, 2 out]
                }
              }
              n138 = property on="is OK?" class="Bool (strict)"("Value"=FALSE ("is OK?")) -> ()  [unwired: 2 in, 2 out]
            }
            frame #1 {
              n139 = while {
                stop <- w138 stop-if-true
                n140 = event shown="[1] \"OK\": Value Change" {
                  selector: _ -> [_ _ _ _ _ _]
                  dyn-events: _ -> [_ _ _ _ _ _]
                  timeout: _ -> [_ _ _ _ _ _]
                  tunnel: [_ TRUE _ TRUE _ _] -> w138
                  event Timeout {
                    n141 = event-data() -> ()  [unwired: 1 in, 2 out]
                  }
                  event "OK": Value Change {
                    n142 = event-data() -> ()  [unwired: 1 in, 5 out]
                    n143 = stacked-sequence {
                      frame #0 {
                        n144 = property on="Al bubbler" class="Clust (strict)"() -> ("Value"=w144:T2)  [unwired: 2 in, 2 out]
                        n145 = Unbundle By Name(w144) -> ("Prep"=w143:bool, "Run"=w142:bool, "Flow"=w141:dbl)
                        n146 = property on="Al Run" class="Bool (strict)"("Value"=w142) -> ()  [unwired: 2 in, 2 out]
                        n147 = property on="Al Prep" class="Bool (strict)"("Value"=w143) -> ()  [unwired: 2 in, 2 out]
                        n148 = property on="Al Flow" class="DigNum (strict)"("Value"=w141) -> ()  [unwired: 2 in, 2 out]
                      }
                      frame #1 {
                        n149 = property on="Ga bubbler" class="Clust (strict)"() -> ("Value"=w153:T1)  [unwired: 2 in, 2 out]
                        n150 = Unbundle By Name(w153) -> ("Prep"=w152:bool, "Run"=w151:bool, "Flow"=w150:dbl, "Dilution"=w149:bool, "Calculated"=w148:u16, "MFC1 flow"=w147:dbl, "MFC2 flow"=w146:dbl, "MFC3 flow"=w145:dbl)
                        n151 = property on="Ga Prep" class="Bool (strict)"("Value"=w152) -> ()  [unwired: 2 in, 2 out]
                        n152 = property on="Ga Run" class="Bool (strict)"("Value"=w151) -> ()  [unwired: 2 in, 2 out]
                        n153 = property on="Ga Flow" class="DigNum (strict)"("Value"=w150) -> ()  [unwired: 2 in, 2 out]
                        n154 = property on="Ga Dilution" class="Bool (strict)"("Value"=w149) -> ()  [unwired: 2 in, 2 out]
                        n155 = property on="Ga Calculated" class="Ring (strict)"("Value"=w148) -> ()  [unwired: 2 in, 2 out]
                        n156 = property on="Ga MFC1 flow" class="DigNum (strict)"("Value"=w147) -> ()  [unwired: 2 in, 2 out]
                        n157 = property on="Ga MFC2 flow" class="DigNum (strict)"("Value"=w146) -> ()  [unwired: 2 in, 2 out]
                        n158 = property on="Ga MFC3 flow" class="DigNum (strict)"("Value"=w145) -> ()  [unwired: 2 in, 2 out]
                      }
                      frame #2 {
                        n159 = property on="In bubbler" class="Clust (strict)"() -> ("Value"=w157:T2)  [unwired: 2 in, 2 out]
                        n160 = Unbundle By Name(w157) -> ("Prep"=w156:bool, "Run"=w155:bool, "Flow"=w154:dbl)
                        n161 = property on="In Prep" class="Bool (strict)"("Value"=w156) -> ()  [unwired: 2 in, 2 out]
                        n162 = property on="In Run" class="Bool (strict)"("Value"=w155) -> ()  [unwired: 2 in, 2 out]
                        n163 = property on="In Flow" class="DigNum (strict)"("Value"=w154) -> ()  [unwired: 2 in, 2 out]
                      }
                      frame #3 {
                        n164 = property on="P gas" class="Clust (strict)"() -> ("Value"=w161:T2)  [unwired: 2 in, 2 out]
                        n165 = Unbundle By Name(w161) -> ("Prep"=w160:bool, "Run"=w159:bool, "Flow"=w158:dbl)
                        n166 = property on="P gas Prep" class="Bool (strict)"("Value"=w160) -> ()  [unwired: 2 in, 2 out]
                        n167 = property on="P gas Run" class="Bool (strict)"("Value"=w159) -> ()  [unwired: 2 in, 2 out]
                        n168 = property on="P gas Flow" class="DigNum (strict)"("Value"=w158) -> ()  [unwired: 2 in, 2 out]
                      }
                      frame #4 {
                        n169 = property on="As gas" class="Clust (strict)"() -> ("Value"=w165:T2)  [unwired: 2 in, 2 out]
                        n170 = Unbundle By Name(w165) -> ("Prep"=w164:bool, "Run"=w163:bool, "Flow"=w162:dbl)
                        n171 = property on="As gas Flow" class="DigNum (strict)"("Value"=w162) -> ()  [unwired: 2 in, 2 out]
                        n172 = property on="As gas Prep" class="Bool (strict)"("Value"=w164) -> ()  [unwired: 2 in, 2 out]
                        n173 = property on="As gas Run" class="Bool (strict)"("Value"=w163) -> ()  [unwired: 2 in, 2 out]
                      }
                      frame #5 {
                        n174 = property on="P bubbler" class="Clust (strict)"() -> ("Value"=w169:T2)  [unwired: 2 in, 2 out]
                        n175 = Unbundle By Name(w169) -> ("Prep"=w168:bool, "Run"=w167:bool, "Flow"=w166:dbl)
                        n176 = property on="P liq Run" class="Bool (strict)"("Value"=w167) -> ()  [unwired: 2 in, 2 out]
                        n177 = property on="P liq Prep" class="Bool (strict)"("Value"=w168) -> ()  [unwired: 2 in, 2 out]
                        n178 = property on="P liq Flow" class="DigNum (strict)"("Value"=w166) -> ()  [unwired: 2 in, 2 out]
                      }
                      frame #6 {
                        n179 = property on="Se bubbler" class="Clust (strict)"() -> ("Value"=w178:T1)  [unwired: 2 in, 2 out]
                        n180 = Unbundle By Name(w178) -> ("Prep"=w177:bool, "Run"=w176:bool, "Flow"=w175:dbl, "Dilution"=w174:bool, "Calculated"=w173:u16, "MFC1 flow"=w172:dbl, "MFC2 flow"=w171:dbl, "MFC3 flow"=w170:dbl)
                        n181 = property on="Se Prep" class="Bool (strict)"("Value"=w177) -> ()  [unwired: 2 in, 2 out]
                        n182 = property on="Se Run" class="Bool (strict)"("Value"=w176) -> ()  [unwired: 2 in, 2 out]
                        n183 = property on="Se Flow" class="DigNum (strict)"("Value"=w175) -> ()  [unwired: 2 in, 2 out]
                        n184 = property on="Se Dilution" class="Bool (strict)"("Value"=w174) -> ()  [unwired: 2 in, 2 out]
                        n185 = property on="Se Calculated" class="Ring (strict)"("Value"=w173) -> ()  [unwired: 2 in, 2 out]
                        n186 = property on="Se MFC1 flow" class="DigNum (strict)"("Value"=w172) -> ()  [unwired: 2 in, 2 out]
                        n187 = property on="Se MFC2 flow" class="DigNum (strict)"("Value"=w171) -> ()  [unwired: 2 in, 2 out]
                        n188 = property on="Se MFC3 flow" class="DigNum (strict)"("Value"=w170) -> ()  [unwired: 2 in, 2 out]
                      }
                    }
                    n189 = property on="is OK?" class="Bool (strict)"("Value"=TRUE ("is OK?")) -> ()  [unwired: 2 in, 2 out]
                  }
                  event "Ga bubbler.Run", "In bubbler.Run", "P gas.Run", "As gas.Run", "P bubbler.Run", "Se bubbler.Run": Value Change {
                    n190 = event-data() -> ()  [unwired: 1 in, 5 out]
                    n191 = control-ref of="source ref array"() -> (w179:refnum<vi>)
                    n192 = for {
                      tunnel: w179 -> [w191]
                      n193 = control-ref of="Al bubbler"() -> (w181:refnum<vi>)
                      n194 = To More Specific Class(target class=w181, reference=w191) -> (specific class reference=w188:refnum<vi>)  [unwired: 1 in, 1 out]
                      n195 = property class="Clust (strict)"(reference=w188) -> ("Controls[]"=w187:refnum<vi>[])  [unwired: 1 in, 2 out]
                      n196 = Index Array(array=w187, index=2) -> (element=w185:refnum<vi>)
                      n197 = control-ref of="Al Run"() -> (w180:refnum<vi>)
                      n198 = To More Specific Class(target class=w180, reference=w185) -> (specific class reference=w184:refnum<vi>, error out=w183:errorcluster)  [unwired: 1 in]
                      n199 = property class="Bool (strict)"(reference=w184, error in=w183) -> ("Value"=w182:bool)  [unwired: 2 out]
                      n200 = Index Array(array=w187, index=1) -> (element=w189:refnum<vi>)
                      n201 = property class="Ctl"(reference=w189, "Visible"=w182) -> ()  [unwired: 1 in, 2 out]
                    }
                  }
                  event "Cancel": Value Change {
                    n202 = event-data() -> ()  [unwired: 1 in, 5 out]
                  }
                  event "Ga bubbler.Calculated", "Ga bubbler.MFC1 flow", "Ga bubbler.MFC2 flow", "Ga bubbler.MFC3 flow", "Ga bubbler.Flow", "Ga bubbler.Dilution": Value Change {
                    n203 = event-data() -> ()  [unwired: 1 in, 5 out]
                    n204 = property on="Dilution" class="Bool (strict)"() -> ("Value"=w193:bool)  [unwired: 2 in, 2 out]
                    n205 = stacked-sequence {
                      tunnel: w193 -> [w194 w204]
                      frame #0 {
                        n206 = case shown="True" w194 {
                          frame False {
                          }
                          frame True {
                            n207 = property on="Flow" class="DigNum (strict)"() -> ("Value"=w202:dbl)  [unwired: 2 in, 2 out]
                            n208 = property on="Calculated" class="Ring (strict)"() -> ("Value"=w203:u16)  [unwired: 2 in, 2 out]
                            n209 = property on="MFC1 flow" class="DigNum (strict)"() -> ("Value"=w201:dbl)  [unwired: 2 in, 2 out]
                            n210 = property on="MFC2 flow" class="DigNum (strict)"() -> ("Value"=w200:dbl)  [unwired: 2 in, 2 out]
                            n211 = property on="MFC3 flow" class="DigNum (strict)"() -> ("Value"=w199:dbl)  [unwired: 2 in, 2 out]
                            n212 = call "dilutionCalc.vi"("Calculated"=w203, "MFC3"=w199, "MFC2"=w200, "MFC1"=w201, "flow"=w202) -> ("MFC3 out"=w195:dbl, "MFC2 out"=w196:dbl, "MFC1 out"=w197:dbl, "flow out"=w198:dbl)  [unwired: 1 in]
                            n213 = property on="MFC1 flow" class="DigNum (strict)"("Value"=w197) -> ()  [unwired: 2 in, 2 out]
                            n214 = property on="Flow" class="DigNum (strict)"("Value"=w198) -> ()  [unwired: 2 in, 2 out]
                            n215 = property on="MFC3 flow" class="DigNum (strict)"("Value"=w195) -> ()  [unwired: 2 in, 2 out]
                            n216 = property on="MFC2 flow" class="DigNum (strict)"("Value"=w196) -> ()  [unwired: 2 in, 2 out]
                          }
                        }
                      }
                      frame #1 {
                        n217 = case shown="False" w204 {
                          frame False {
                            n218 = property on="Flow" class="DigNum (strict)"("DisabledEnum"=T6."Enabled" ("Disabled")) -> ()  [unwired: 2 in, 2 out]
                          }
                          frame True {
                            n219 = property on="Calculated" class="Ring (strict)"() -> ("Value"=w206:u16)  [unwired: 2 in, 2 out]
                            n220 = call "DilutionVisible.vi"("calculated"=w206) -> ("MFC3"=w210:u16, "MFC2"=w209:u16, "MFC1"=w208:u16, "flow"=w207:u16)  [unwired: 3 in]
                            n221 = property on="MFC1 flow" class="DigNum (strict)"("DisabledEnum"=w208) -> ()  [unwired: 2 in, 2 out]
                            n222 = property on="MFC2 flow" class="DigNum (strict)"("DisabledEnum"=w209) -> ()  [unwired: 2 in, 2 out]
                            n223 = property on="MFC3 flow" class="DigNum (strict)"("DisabledEnum"=w210) -> ()  [unwired: 2 in, 2 out]
                            n224 = property on="Flow" class="DigNum (strict)"("DisabledEnum"=w207) -> ()  [unwired: 2 in, 2 out]
                          }
                        }
                        n225 = property on="Calculated" class="Ring (strict)"("Visible"=w204) -> ()  [unwired: 2 in, 2 out]
                        n226 = property on="MFC1 flow" class="DigNum (strict)"("Visible"=w204) -> ()  [unwired: 2 in, 2 out]
                        n227 = property on="MFC2 flow" class="DigNum (strict)"("Visible"=w204) -> ()  [unwired: 2 in, 2 out]
                        n228 = property on="MFC3 flow" class="DigNum (strict)"("Visible"=w204) -> ()  [unwired: 2 in, 2 out]
                      }
                    }
                  }
                  event "Se bubbler.MFC1 flow", "Se bubbler.MFC3 flow", "Se bubbler.MFC2 flow", "Se bubbler.Flow", "Se bubbler.Calculated", "Se bubbler.Dilution": Value Change {
                    n229 = event-data() -> ()  [unwired: 1 in, 5 out]
                    n230 = property on="Dilution" class="Bool (strict)"() -> ("Value"=w211:bool)  [unwired: 2 in, 2 out]
                    n231 = stacked-sequence {
                      tunnel: w211 -> [w212 w222]
                      frame #0 {
                        n232 = case shown="True" w212 {
                          frame False {
                          }
                          frame True {
                            n233 = property on="Flow" class="DigNum (strict)"() -> ("Value"=w220:dbl)  [unwired: 2 in, 2 out]
                            n234 = property on="Calculated" class="Ring (strict)"() -> ("Value"=w221:u16)  [unwired: 2 in, 2 out]
                            n235 = property on="MFC1 flow" class="DigNum (strict)"() -> ("Value"=w219:dbl)  [unwired: 2 in, 2 out]
                            n236 = property on="MFC2 flow" class="DigNum (strict)"() -> ("Value"=w218:dbl)  [unwired: 2 in, 2 out]
                            n237 = property on="MFC3 flow" class="DigNum (strict)"() -> ("Value"=w217:dbl)  [unwired: 2 in, 2 out]
                            n238 = call "dilutionCalc.vi"("Calculated"=w221, "MFC3"=w217, "MFC2"=w218, "MFC1"=w219, "flow"=w220) -> ("MFC3 out"=w213:dbl, "MFC2 out"=w214:dbl, "MFC1 out"=w215:dbl, "flow out"=w216:dbl)  [unwired: 1 in]
                            n239 = property on="MFC1 flow" class="DigNum (strict)"("Value"=w215) -> ()  [unwired: 2 in, 2 out]
                            n240 = property on="Flow" class="DigNum (strict)"("Value"=w216) -> ()  [unwired: 2 in, 2 out]
                            n241 = property on="MFC3 flow" class="DigNum (strict)"("Value"=w213) -> ()  [unwired: 2 in, 2 out]
                            n242 = property on="MFC2 flow" class="DigNum (strict)"("Value"=w214) -> ()  [unwired: 2 in, 2 out]
                          }
                        }
                      }
                      frame #1 {
                        n243 = case shown="True" w222 {
                          frame False {
                            n244 = property on="Flow" class="DigNum (strict)"("DisabledEnum"=T6."Enabled" ("Disabled")) -> ()  [unwired: 2 in, 2 out]
                          }
                          frame True {
                            n245 = property on="Calculated" class="Ring (strict)"() -> ("Value"=w224:u16)  [unwired: 2 in, 2 out]
                            n246 = call "DilutionVisible.vi"("calculated"=w224) -> ("MFC3"=w228:u16, "MFC2"=w227:u16, "MFC1"=w226:u16, "flow"=w225:u16)  [unwired: 3 in]
                            n247 = property on="MFC1 flow" class="DigNum (strict)"("DisabledEnum"=w226) -> ()  [unwired: 2 in, 2 out]
                            n248 = property on="MFC2 flow" class="DigNum (strict)"("DisabledEnum"=w227) -> ()  [unwired: 2 in, 2 out]
                            n249 = property on="MFC3 flow" class="DigNum (strict)"("DisabledEnum"=w228) -> ()  [unwired: 2 in, 2 out]
                            n250 = property on="Flow" class="DigNum (strict)"("DisabledEnum"=w225) -> ()  [unwired: 2 in, 2 out]
                          }
                        }
                        n251 = property on="Calculated" class="Ring (strict)"("Visible"=w222) -> ()  [unwired: 2 in, 2 out]
                        n252 = property on="MFC1 flow" class="DigNum (strict)"("Visible"=w222) -> ()  [unwired: 2 in, 2 out]
                        n253 = property on="MFC2 flow" class="DigNum (strict)"("Visible"=w222) -> ()  [unwired: 2 in, 2 out]
                        n254 = property on="MFC3 flow" class="DigNum (strict)"("Visible"=w222) -> ()  [unwired: 2 in, 2 out]
                      }
                    }
                  }
                }
              }
            }
            frame #2 {
              n255 = property on="is OK?" class="Bool (strict)"() -> ("Value"=w229:bool)  [unwired: 2 in, 2 out]
              n256 = Not(x=w229) -> (.not. x?=w233:bool)
              n257 = Current VI's Path() -> (path=w232:path)
              n258 = call "API_Edit.vi"("Cancel"=w233, "OK"=w229, "VI Path"=w232, "Argument List In"=w230) -> ("Argument List Out"=w231:string[])
            }
          }
          n259 = property class="VI"(reference=w106, "Front Panel.Open"=FALSE ("Front Panel Window:Open"), "FP.Behavior"=T5."Default" ("Front Panel Window:Behavior")) -> (reference out=w107:refnum<vi>)  [unwired: 1 in, 1 out]
          n260 = Close Reference(reference=w107) -> ()  [unwired: 1 in, 1 out]
        }
        frame "Start" {
          n261 = call "Set_Argument.vi"("Enable"=FALSE, "Argument"="run_started", "Argument List In"=w240) -> ("Argument List Out"=w239:string[])
          n262 = property on="prep_time" class="DigNum (strict)"() -> ("Value"=w238:dbl)  [unwired: 2 in, 2 out]
          n263 = Greater Than 0?(x=w238) -> (x > 0?=w237:bool)
          n264 = Not(x=w235) -> (.not. x?=w234:bool)
          n265 = And(x=w234, y=w237) -> (x .and. y?=w236:bool)
          n266 = case shown="True" w236 {
            frame False {
            }
            frame True {
              n267 = property on="Al bubbler" class="Clust (strict)"() -> ("Value"=w243:T2)  [unwired: 2 in, 2 out]
              n268 = call "Set_V_III.vi"("Run Started"=FALSE, "Al bubbler"=w243) -> ()  [unwired: 10 in]
            }
          }
        }
        frame "Run" {
          n269 = stacked-sequence {
            tunnel: w248 -> [_ w253 _ _]
            tunnel: w246 -> [w250 _ _ w327]
            tunnel: w247 -> [_ _ _ w325]
            tunnel: [_ _ _ w326] -> w245
            frame #0 {
              n270 = call "Get_Argument.vi"("Argument"="run_started", "Argument List"=w250) -> ("Enabled"=w249:bool)
              n271 = local write "run started"(w249) -> ()
            }
            frame #1 {
              n272 = property on="prep_time" class="DigNum (strict)"() -> ("Value"=w254:dbl)  [unwired: 2 in, 2 out]
              n273 = Greater Or Equal?(x=w253, y=w254) -> (x >= y?=w252:bool)
              n274 = local write "prep_done"(w252) -> ()
            }
            frame #2 {
              n275 = local read "run started"() -> (w256:bool)
              n276 = Not(x=w256) -> (.not. x?=w255:bool)
              n277 = stacked-sequence {
                tunnel: w255 -> [w258 w264 w273 w282 w291 w300 w309 w318]
                frame #0 {
                  n278 = case shown="False" w258 {
                    tunnel: ["run: " "pre-run: "] -> w257
                    frame False {
                    }
                    frame True {
                    }
                  }
                  n279 = property on="Status Out" class="Str"("Value"=w257) -> ()  [unwired: 2 in, 2 out]
                }
                frame #1 {
                  n280 = property on="Active" class="Bool (strict)"() -> ("Value"=w263:bool)  [unwired: 2 in, 2 out]
                  n281 = property on="Status Out" class="Str"() -> ("Value"=w269:string)  [unwired: 2 in, 2 out]
                  n282 = Unbundle By Name() -> ("Al Run"=w262:bool, "Prep Al"=w261:bool)  [unwired: 1 in]
                  n283 = call "flow_strings.vi"("string in"=w269, "is first in?"=TRUE, "use source?"=w263, "name"="Al", "run source?"=w262, "prep source?"=w261, "is prep?"=w264) -> ("string out"=w268:string, "is first out?"=w267:bool)
                  n284 = property on="Status Out" class="Str"("Value"=w268) -> ()  [unwired: 2 in, 2 out]
                  n285 = property on="first" class="Bool (strict)"("Value"=w267) -> ()  [unwired: 2 in, 2 out]
                }
                frame #2 {
                  n286 = property on="Ga bubbler" class="Clust (strict)"() -> ("Value"=w272:T1)  [unwired: 2 in, 2 out]
                  n287 = property on="first" class="Bool (strict)"() -> ("Value"=w275:bool)  [unwired: 2 in, 2 out]
                  n288 = property on="Status Out" class="Str"() -> ("Value"=w277:string)  [unwired: 2 in, 2 out]
                  n289 = Unbundle By Name(w272) -> ("Run"=w271:bool, "Prep"=w270:bool)
                  n290 = call "flow_strings.vi"("string in"=w277, "is first in?"=w275, "name"="Ga", "run source?"=w271, "prep source?"=w270, "is prep?"=w273) -> ("string out"=w278:string, "is first out?"=w274:bool)  [unwired: 1 in]
                  n291 = property on="Status Out" class="Str"("Value"=w278) -> ()  [unwired: 2 in, 2 out]
                  n292 = property on="first" class="Bool (strict)"("Value"=w274) -> ()  [unwired: 2 in, 2 out]
                }
                frame #3 {
                  n293 = property on="In bubbler" class="Clust (strict)"() -> ("Value"=w281:T2)  [unwired: 2 in, 2 out]
                  n294 = property on="first" class="Bool (strict)"() -> ("Value"=w285:bool)  [unwired: 2 in, 2 out]
                  n295 = property on="Status Out" class="Str"() -> ("Value"=w287:string)  [unwired: 2 in, 2 out]
                  n296 = Unbundle By Name(w281) -> ("Run"=w280:bool, "Prep"=w279:bool)
                  n297 = call "flow_strings.vi"("string in"=w287, "is first in?"=w285, "name"="In", "run source?"=w280, "prep source?"=w279, "is prep?"=w282) -> ("string out"=w284:string, "is first out?"=w283:bool)  [unwired: 1 in]
                  n298 = property on="Status Out" class="Str"("Value"=w284) -> ()  [unwired: 2 in, 2 out]
                  n299 = property on="first" class="Bool (strict)"("Value"=w283) -> ()  [unwired: 2 in, 2 out]
                }
                frame #4 {
                  n300 = property on="P gas" class="Clust (strict)"() -> ("Value"=w290:T2)  [unwired: 2 in, 2 out]
                  n301 = property on="first" class="Bool (strict)"() -> ("Value"=w293:bool)  [unwired: 2 in, 2 out]
                  n302 = property on="Status Out" class="Str"() -> ("Value"=w295:string)  [unwired: 2 in, 2 out]
                  n303 = Unbundle By Name(w290) -> ("Run"=w289:bool, "Prep"=w288:bool)
                  n304 = call "flow_strings.vi"("string in"=w295, "is first in?"=w293, "name"="PH3", "run source?"=w289, "prep source?"=w288, "is prep?"=w291) -> ("string out"=w294:string, "is first out?"=w292:bool)  [unwired: 1 in]
                  n305 = property on="Status Out" class="Str"("Value"=w294) -> ()  [unwired: 2 in, 2 out]
                  n306 = property on="first" class="Bool (strict)"("Value"=w292) -> ()  [unwired: 2 in, 2 out]
                }
                frame #5 {
                  n307 = property on="As gas" class="Clust (strict)"() -> ("Value"=w299:T2)  [unwired: 2 in, 2 out]
                  n308 = property on="first" class="Bool (strict)"() -> ("Value"=w302:bool)  [unwired: 2 in, 2 out]
                  n309 = property on="Status Out" class="Str"() -> ("Value"=w304:string)  [unwired: 2 in, 2 out]
                  n310 = Unbundle By Name(w299) -> ("Run"=w298:bool, "Prep"=w297:bool)
                  n311 = call "flow_strings.vi"("string in"=w304, "is first in?"=w302, "name"="AsH3", "run source?"=w298, "prep source?"=w297, "is prep?"=w300) -> ("string out"=w301:string, "is first out?"=w303:bool)  [unwired: 1 in]
                  n312 = property on="Status Out" class="Str"("Value"=w301) -> ()  [unwired: 2 in, 2 out]
                  n313 = property on="first" class="Bool (strict)"("Value"=w303) -> ()  [unwired: 2 in, 2 out]
                }
                frame #6 {
                  n314 = property on="P bubbler" class="Clust (strict)"() -> ("Value"=w308:T2)  [unwired: 2 in, 2 out]
                  n315 = property on="first" class="Bool (strict)"() -> ("Value"=w312:bool)  [unwired: 2 in, 2 out]
                  n316 = property on="Status Out" class="Str"() -> ("Value"=w314:string)  [unwired: 2 in, 2 out]
                  n317 = Unbundle By Name(w308) -> ("Run"=w307:bool, "Prep"=w306:bool)
                  n318 = call "flow_strings.vi"("string in"=w314, "is first in?"=w312, "name"="P liq", "run source?"=w307, "prep source?"=w306, "is prep?"=w309) -> ("string out"=w311:string, "is first out?"=w310:bool)  [unwired: 1 in]
                  n319 = property on="Status Out" class="Str"("Value"=w311) -> ()  [unwired: 2 in, 2 out]
                  n320 = property on="first" class="Bool (strict)"("Value"=w310) -> ()  [unwired: 2 in, 2 out]
                }
                frame #7 {
                  n321 = property on="Se bubbler" class="Clust (strict)"() -> ("Value"=w317:T1)  [unwired: 2 in, 2 out]
                  n322 = property on="first" class="Bool (strict)"() -> ("Value"=w321:bool)  [unwired: 2 in, 2 out]
                  n323 = property on="Status Out" class="Str"() -> ("Value"=w323:string)  [unwired: 2 in, 2 out]
                  n324 = Unbundle By Name(w317) -> ("Run"=w316:bool, "Prep"=w315:bool)
                  n325 = call "flow_strings.vi"("string in"=w323, "is first in?"=w321, "name"="Se", "run source?"=w316, "prep source?"=w315, "is prep?"=w318) -> ("string out"=w320:string, "is first out?"=w319:bool)  [unwired: 1 in]
                  n326 = property on="Status Out" class="Str"("Value"=w320) -> ()  [unwired: 2 in, 2 out]
                  n327 = property on="first" class="Bool (strict)"("Value"=w319) -> ()  [unwired: 2 in, 2 out]
                }
              }
            }
            frame #3 {
              n328 = property on="prep_done" class="Bool (strict)"() -> ("Value"=w330:bool)  [unwired: 2 in, 2 out]
              n329 = property on="run started" class="Bool (strict)"() -> ("Value"=w329:bool)  [unwired: 2 in, 2 out]
              n330 = Not(x=w329) -> (.not. x?=w328:bool)
              n331 = And(x=w330, y=w328) -> (x .and. y?=w324:bool)
              n332 = case shown="True" w324 {
                selector: w324 -> [_ w332]
                tunnel: w327 -> [w331 w335]
                tunnel: [w331 w334] -> w326
                tunnel: w325 -> [_ w333]
                frame False {
                }
                frame True {
                  n333 = stacked-sequence {
                    tunnel: w333 -> [w337 _]
                    tunnel: w335 -> [_ w340]
                    tunnel: [_ w339] -> w334
                    tunnel: w332 -> [w336 _]
                    frame #0 {
                      n334 = case shown="False" w337 {
                        tunnel: w336 -> [w338 _]
                        frame False {
                          n335 = call "Set_V_III.vi"("Run Started"=w338) -> ()  [unwired: 11 in]
                        }
                        frame True {
                        }
                      }
                    }
                    frame #1 {
                      n336 = call "Set_Argument.vi"("Enable"=TRUE, "Argument"="run_started", "Argument List In"=w340) -> ("Argument List Out"=w339:string[])
                    }
                  }
                }
              }
            }
          }
        }
        frame "End" {
        }
        frame "Idle" {
        }
      }
    }
  }
  "Argument List Out" <- w10
